vi "Read All Table Data.vi"(8 "error in (no error)":errorcluster) -> (0 "error out":errorcluster)   [LabVIEW 2020, in "Settings.lvlib"]
uses:
  Settings.lvlib
  <vilib>/drjdpowell/SQLite Library/SQL Connection/Open (path).vi
  <vilib>/drjdpowell/SQLite Library/SQL Connection/Open (string).vi
  <vilib>/AdvancedString/Path To Command Line String.vi
  <vilib>/drjdpowell/SQLite Library/SQL Connection/Execute SQL.vi
  <vilib>/drjdpowell/SQLite Library/SQL Connection/Connection.lvclass
  <vilib>/drjdpowell/SQLite Library/SQLite.lvlib
panel:
  out "Tasks Appended":string[][](array[string])
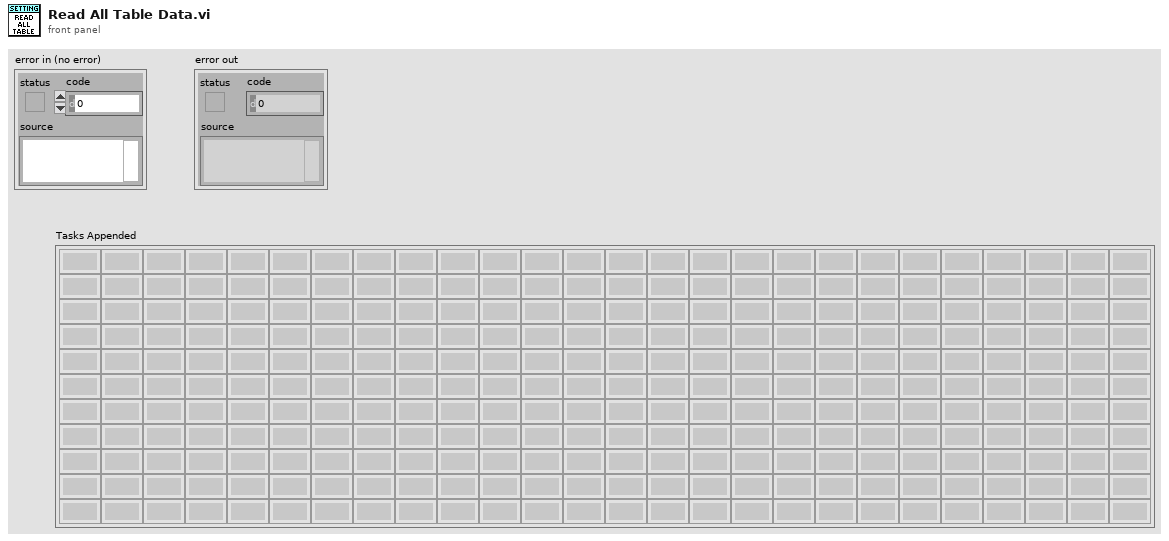
[diagram p1: front panel]
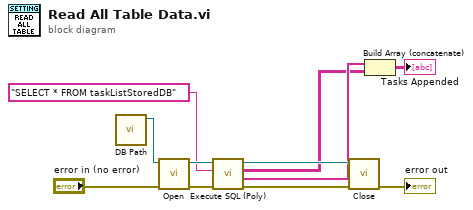
[diagram p0: block diagram]
diagram:
  n1 = call "DB Path.vi"() -> ("DB Path"=w6:path)  [unwired: 11 in]
  n2 = call-poly <vilib>:"Open.vi"("error in (no error)"="error in (no error)", "db file"=w6) -> ("error out"=w11:errorcluster, "SQLite Connection"=w9:refnum<class "Connection.lvclass">)  [unwired: 8 in]
  n3 = call-poly <vilib>:"Execute SQL (Poly).vi"("error in (no error)"=w11, "SQL"="SELECT * FROM taskListStoredDB", "SQLite Connection in"=w9) -> ("error out"=w10:errorcluster, "Column Names"=w3:string[], "Result Set"=w1:string[][], "SQLite Connection"=w8:refnum<class "Connection.lvclass">)  [unwired: 5 in]
  n4 = call-dynamic "Close.vi"("error in (no error)"=w10, "SQLite Connection in"=w8) -> ("error out"=→"error out":errorcluster)  [unwired: 9 in]
  n5 = Build Array (concatenate)(w3, w1) -> (→"Tasks Appended":string[][])
